vi "initial test.vi"() -> ()   [LabVIEW 2020]
panel:
  out "|Z|":dbl
  out "Impedance":cdb
  out "START":cdb
  out "loss db":dbl
  out "degree":dbl
  out "Magnitude":dbl
  out "theta":dbl
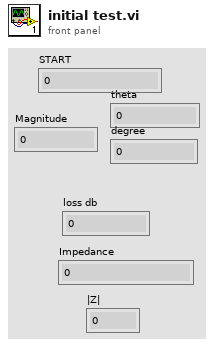
[diagram p1: front panel]
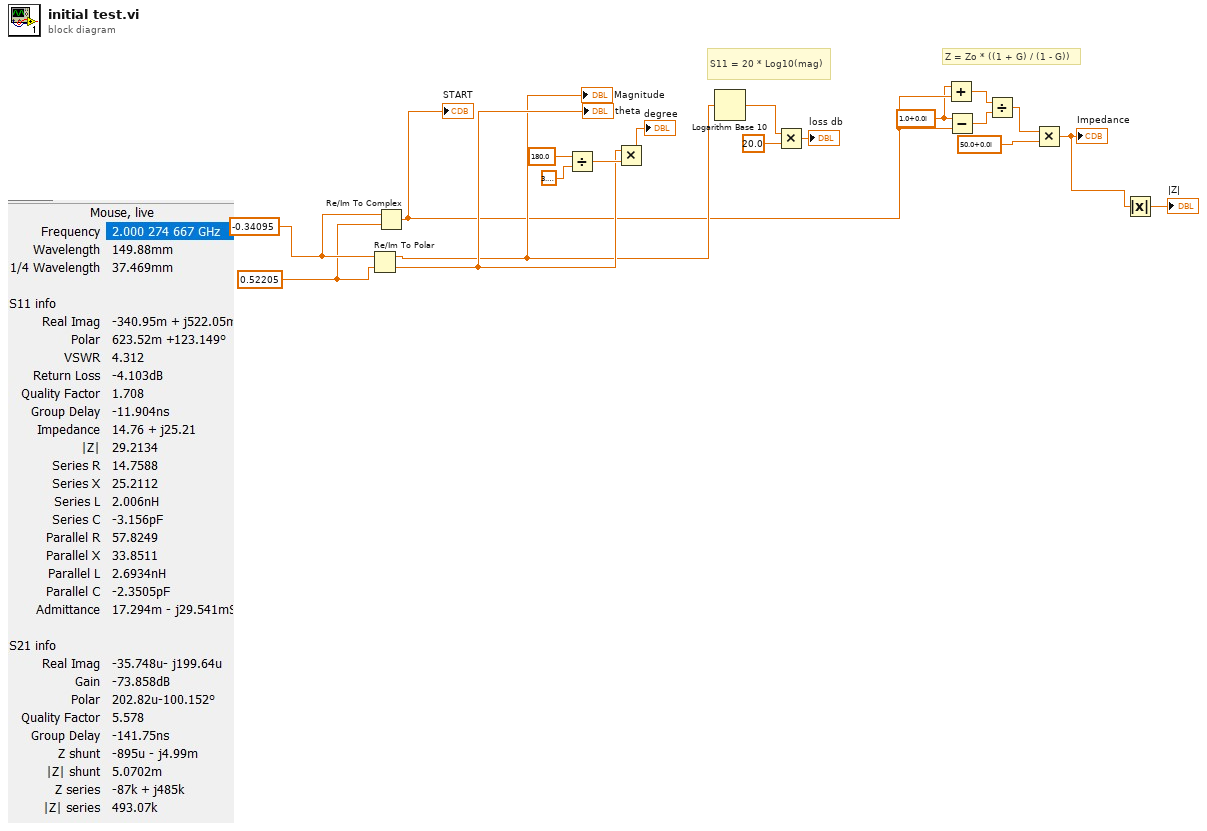
[diagram p0: block diagram]
diagram:
  w7 = cdb 1.0+0.0i ("x")
  w11 = 0.52205 ("x")
  w12 = -0.34095 ("x")
  # "Z = Zo * ((1 + G) / (1 - G))"
  # "S11 = 20 * Log10(mag)"
  n1 = Re/Im To Polar(2:w11, 3:w12) -> (0:w10:dbl, 1:w9:dbl)
  "theta" <- w10
  "Magnitude" <- w9
  n2 = Re/Im To Complex(1:w11, 2:w12) -> (0:w8:cdb)
  "START" <- w8
  n3 = Divide(x=180.0, y=3.141592653589793) -> (x/y=w17:dbl)
  n4 = Multiply(x=w10, y=w17) -> (x*y=→"degree":dbl)
  n5 = Logarithm Base 10(1:w9) -> (0:w15:dbl)
  n6 = Multiply(x=w15, y=20.0) -> (x*y=→"loss db":dbl)
  n7 = Add(x=w7, y=w8) -> (x+y=w6:cdb)
  n8 = Subtract(x=w7, y=w8) -> (x-y=w5:cdb)
  n9 = Divide(x=w6, y=w5) -> (x/y=w4:cdb)
  n10 = Multiply(x=w4, y=cdb 50.0+0.0i) -> (x*y=w2:cdb)
  "Impedance" <- w2
  n11 = Absolute Value(x=w2) -> (abs(x)=→"|Z|":dbl)
